vi "Set Tag Protocol.vi"(8 "error in (no error)":errorcluster, 9 "Protocol":u8=5 format="%x", 10 "Baud Rate":u32=38400, 11 "COM Port":refnum<visa-resource-name>="COM4") -> (0 "error out":errorcluster, 2 "received str":string, 3 "Result":bool)   [LabVIEW 2018]
panel:
  # "SET TAG PROTOCOL"
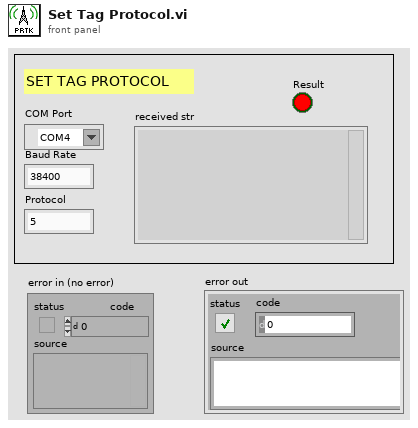
[diagram p1: front panel]
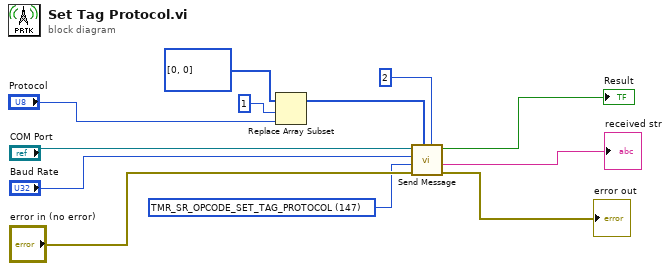
[diagram p0: block diagram]
diagram:
  w1 = u16 147 items=["TMR_SR_OPCODE_VERSION"=3, "TMR_SR_OPCODE_SET_BAUD_RATE"=6, "TMR_SR_OPCODE_READ_TAG_ID_SINGLE"=33, "TMR_SR_OPCODE_READ_TAG_ID_MULTIPLE"=34, "TMR_SR_OPCODE_WRITE_TAG_ID"=35, "TMR_SR_OPCODE_WRITE_TAG_DATA"=36, "TMR_SR_OPCODE_KILL_TAG"=38, "TMR_SR_OPCODE_READ_TAG_DATA"=40, "TMR_SR_OPCODE_CLEAR_TAG_ID_BUFFER"=42, "TMR_SR_OPCODE_MULTI_PROTOCOL_TAG_OP"=47, "TMR_SR_OPCODE_GET_READ_TX_POWER"=98, "TMR_SR_OPCODE_GET_WRITE_TX_POWER"=100, "TMR_SR_OPCODE_GET_POWER_MODE"=104, "TMR_SR_OPCODE_GET_READER_OPTIONAL_PARAMS"=106, "TMR_SR_OPCODE_GET_PROTOCOL_PARAM"=107, "TMR_SR_OPCODE_SET_ANTENNA_PORT"=145, "TMR_SR_OPCODE_SET_TAG_PROTOCOL"=147, "TMR_SR_OPCODE_SET_READ_TX_POWER"=146, "TMR_SR_OPCODE_SET_WRITE_TX_POWER"=148, "TMR_SR_OPCODE_SET_REGION"=151, "TMR_SR_OPCODE_SET_READER_OPTIONAL_PARAMS"=154, "TMR_SR_OPCODE_SET_PROTOCOL_PARAM"=155] ("Opcode Constant")
  n1 = Replace Array Subset(array=u8[] [0, 0], new element="Protocol", index=1) -> (w7:u8[])
  n2 = call "Send Message.vi"("Size"=u8 2, "Data"=w7, "error in (no error)"="error in (no error)", "Opcode"=w1, "Baud Rate"="Baud Rate", "COM Port"="COM Port") -> ("error out"=→"error out":errorcluster, "received str"=→"received str":string, "Result"=→"Result":bool)  [unwired: 2 in, 1 out]
